vi "XYStage.GetPublicEventsRegistration.vi"(8 "error in (no error)":errorcluster, 11 "XYStage":refnum<class "XYStage.lvclass">) -> (0 "error out":errorcluster, 2 "XYStage Public Events":refnum<event-registration>, 3 "XYStage out":refnum<class "XYStage.lvclass">)   [LabVIEW 2017, in "XYStage.lvclass"]
doc: "---------------------------------------------------------------\nJKI State Machine Objects™\nhttp://jki.net/state-machine-objects/\nCopyright (C) 2005-2015, JKI <info@jki.net>\nALL RIGHTS RESERVEDJKI State Machine Objects (SMO) 1.0.0.5\nJKI - JKI\nCopyright (c) 2016, JKI"
uses:
  XYStage.lvclass
  Typedefs/PublicEvents--Cluster.ctl
  Typedefs/PublicEvents--XYStage.MoveStarted.ctl
  Typedefs/Coordinates--Cluster.ctl
  Typedefs/Coordinates.Units--Cluster.ctl
  Typedefs/Coordinates.Counts--Cluster.ctl
  Typedefs/PublicEvents--XYStage.MoveCompleted.ctl
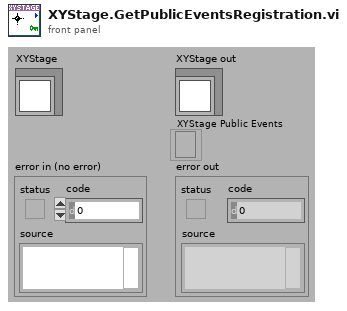
[diagram p1: front panel]
types:
  T1 = typedef "XYStage.lvclass/PublicEvents--Cluster.ctl" = cluster{"MoveStarted":refnum<user-event>, "MoveCompleted":refnum<user-event>}
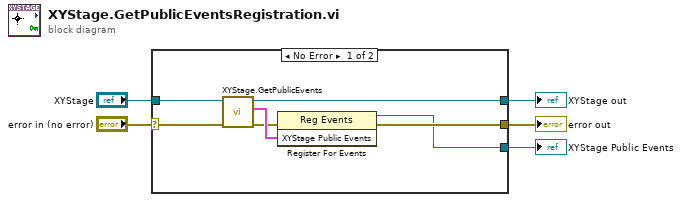
[diagram p0: block diagram]
diagram:
  n1 = case shown="No Error" "error in (no error)" {
    selector: "error in (no error)" -> [w6 w13]
    tunnel: "XYStage" -> [w11 w14]
    tunnel: [w9 w13] -> w4
    tunnel: [w10 w14] -> w3
    tunnel: [w8 _] -> w1
    frame No Error {
      n2 = call "XYStage.GetPublicEvents.vi"("error in (no error)"=w6, "XYStage"=w11) -> ("error out"=w7:errorcluster, "XYStage Public Events"=w12:T1, "XYStage out"=w10:refnum<class "XYStage.lvclass">)  [unwired: 7 in]
      n3 = register-events(error in=w7, w12) -> (reference out=w8:refnum<event-registration>, error out=w9:errorcluster)  [unwired: 1 in]
    }
    frame Error {
    }
  }
  "error out" <- w4
  "XYStage out" <- w3
  "XYStage Public Events" <- w1
